vi "generate_single_vi.vi"(8 "error in (no error)":errorcluster, 11 "Single VI Spec":T1={"Configure Specs In"=[{"Instrument Command"=":SYST%s:PON:TYPE %s;", "Controls Specs"=[{"Control Label"="ring0", "Control Data Type"=enum."I32", "Control Class"=enum."Text Ring", "BD Text"="1\n2\n3\n4", "Ring Strings and Values"=[{"String"="1", "Value"=0.0}, {"String"="2", "Value"=1.0}, {"String"="3", "Value"=2.0}, {"String"="4", "Value"=3.0}], "Required Input"=FALSE, "Default Value"="0"}, {"Control Label"="ring1", "Control Data Type"=enum."I32", "Control Class"=enum."Text Ring", "BD Text"="MODE\nUSER\nLAST\nPRES", "Ring Strings and Values"=[{"String"="MODE", "Value"=0.0}, {"String"="USER", "Value"=1.0}, {"String"="LAST", "Value"=2.0}, {"String"="PRES", "Value"=3.0}], "Required Input"=FALSE, "Default Value"="0"}]}], "VI Paths"=path "c:/Users/hachen/Desktop/test.vi", "Control Label Sequences"=[]}) -> (0 "error out":errorcluster)   [LabVIEW 2018]
uses:
  TypeDefinitions/single_vi_spec.ctl
  TypeDefinitions/single_cmd_spec.ctl
  TypeDefinitions/single_control_spec.ctl
  TypeDefinitions/control_data_type.ctl
  TypeDefinitions/control_class.ctl
  TypeDefinitions/ring_string_and_value.ctl
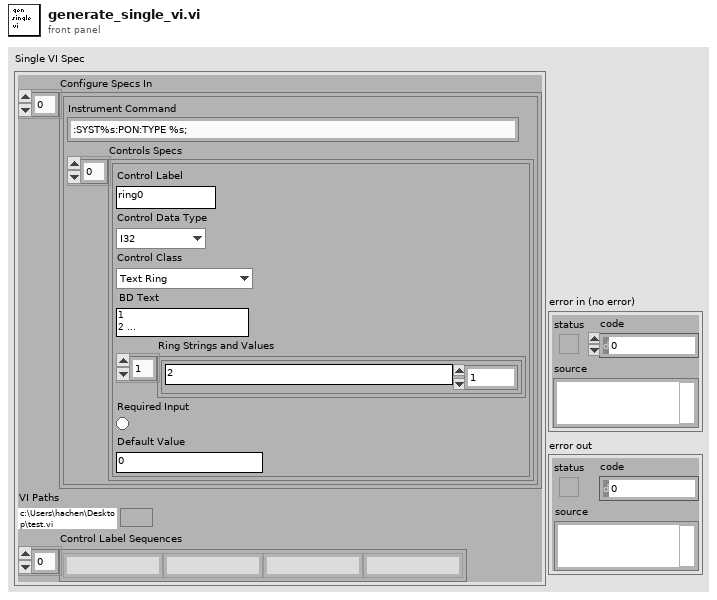
[diagram p1: front panel]
types:
  T1 = typedef "single_vi_spec.ctl" = cluster{"Configure Specs In":T2[], "VI Paths":path, "Control Label Sequences":string[]}
  T2 = typedef "single_cmd_spec.ctl" = cluster{"Instrument Command":string, "Controls Specs":T3[]}
  T3 = typedef "single_control_spec.ctl" = cluster{"Control Label":string, "Control Data Type":T4, "Control Class":T5, "BD Text":string, "Ring Strings and Values":T6[], "Required Input":bool, "Default Value":string}
  T4 = typedef "control_data_type.ctl" = enum16{"DBL", "I32", "Boolean", "String", "U16", "U32", "EXT", "SGL", "I16", "U8", "I8", "I64", "U64", "Waveform", "Reference", "Variant", "Cluster"}
  T5 = typedef "control_class.ctl" = enum16{"Numeric", "Vertical Slide Switch", "Text Ring", "String", "Array", "VISAName", "WaveformGraph", "Cluster"}
  T6 = typedef "ring_string_and_value.ctl" = cluster{"String":string, "Value":dbl}
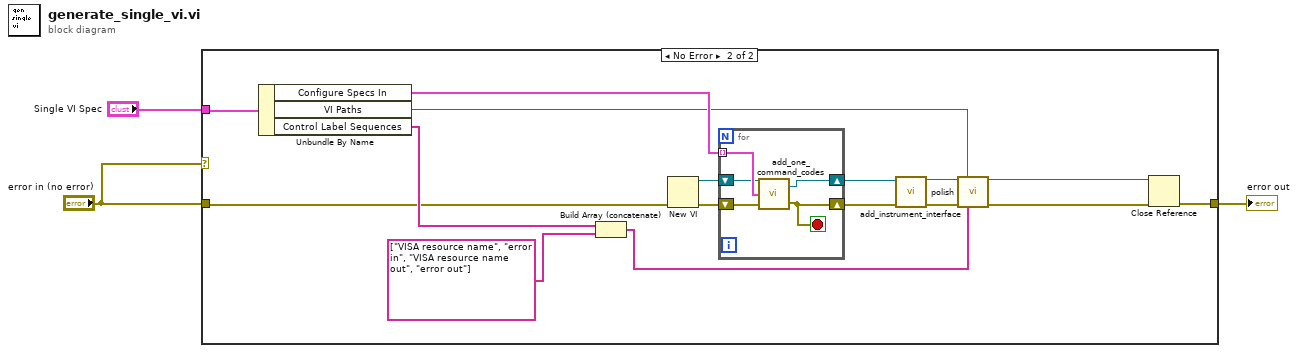
[diagram p0: block diagram]
diagram:
  n1 = case shown="No Error" "error in (no error)" {
    tunnel: [w4 w5] -> w3
    tunnel: "error in (no error)" -> [w4 w6]
    tunnel: "Single VI Spec" -> [_ w7]
    frame Error {
    }
    frame No Error {
      n2 = Unbundle By Name(w7) -> ("Configure Specs In"=w12:T2[], "VI Paths"=w10:path, "Control Label Sequences"=w18:string[])
      n3 = Build Array (concatenate)(w18, string[] ["VISA resource name", "error in", "VISA resource name out", "error out"] ("element")) -> (w16:string[])
      n4 = New VI(8:w6) -> (0:w19:errorcluster, 3:w15:refnum<vi>)  [unwired: 1 in, 5 out]
      n5 = for {
        shift-right: [w23] -> w11
        shift-left: w15 -> [w24]
        tunnel: w12 -> [w25] mode=indexing
        shift-right: [w21] -> w20
        shift-left: w19 -> [w22]
        stop <- w21 stop-if-true
        n6 = call "add_one_command_codes.vi"("error in"=w22, "Single Command Spec"=w25, "VI Ref In"=w24) -> ("error out"=w21:errorcluster, "VI Ref Out"=w23:refnum<vi>)
      }
      n7 = call "add_instrument_interface.vi"("VI Ref In"=w11, "error in"=w20) -> ("VI Ref Out"=w8:refnum<vi>, "error out"=w9:errorcluster)  [unwired: 5 in, 7 out]
      n8 = call "polish.vi"("VI Ref In"=w8, "VI Path"=w10, "error in"=w9, "Ctrl Sequences"=w16) -> ("VI Ref Out"=w14:refnum<vi>, "error out"=w13:errorcluster)  [unwired: 3 in, 7 out]
      n9 = Close Reference(reference=w14, error in (no error)=w13) -> (error out=w5:errorcluster)
    }
  }
  "error out" <- w3
